vi "Create Encryption.vi"(6 "Multiplier":dbl, 8 "Error In":errorcluster, 9 "SALT location (start of string)":u16(ring)=1 items=["both", "start of string", "end of string"], 10 "SALT":string, 11 "Encryption Method":refnum<class "Encryption.lvclass">) -> (0 "Error Out":errorcluster, 3 "Encryption output":refnum<class "Encryption.lvclass">)   [LabVIEW 2019, in "TSC Event Logger.lvlib" / "Encryption.lvclass"]
uses:
  Encryption.lvclass
  Encryption.lvclass/Encryption.ctl
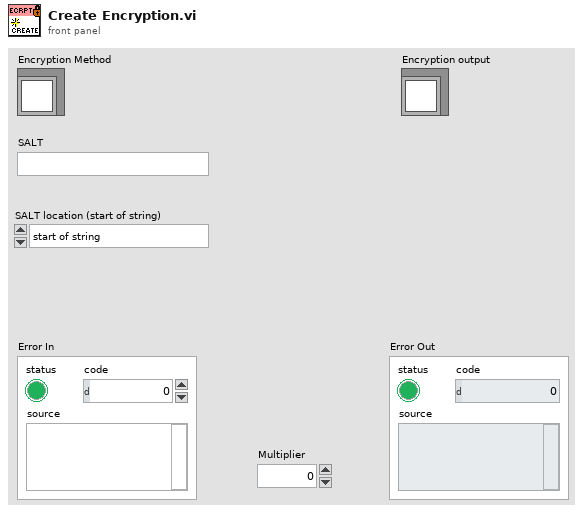
[diagram p1: front panel]
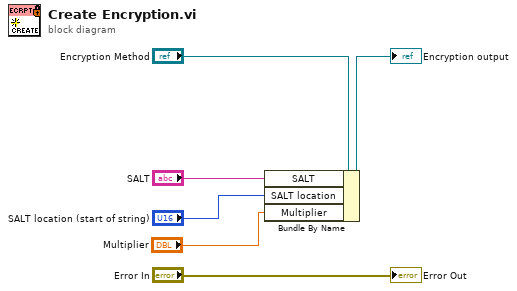
[diagram p0: block diagram]
diagram:
  n1 = Bundle By Name(cluster="Encryption Method", "SALT"="SALT", "SALT location"="SALT location (start of string)", "Multiplier"="Multiplier") -> (→"Encryption output":refnum<class "Encryption.lvclass">)
  "Error Out" <- "Error In"
